vi "findValue.vi"(1 "采集数据":dbl[](array[numeric]), 2 "精度":dbl, 3 "循环点":i32) -> (0 "试验结果":dbl[](array[numeric]))   [LabVIEW 2011]
panel:
  out "内部变量":i32
  out "Numeric":dbl
  out "标志":bool
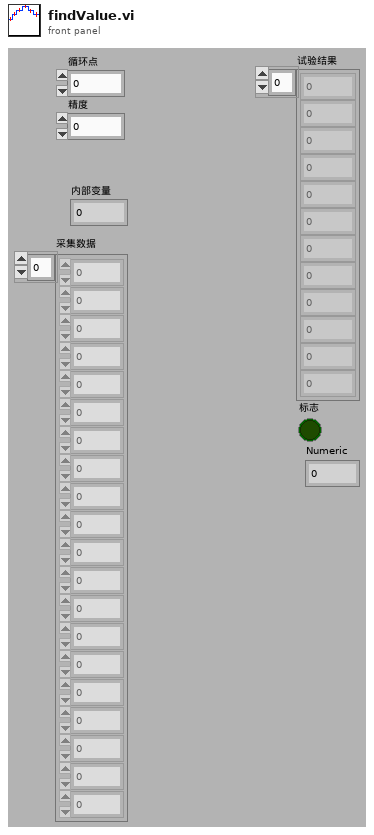
[diagram p1: front panel]
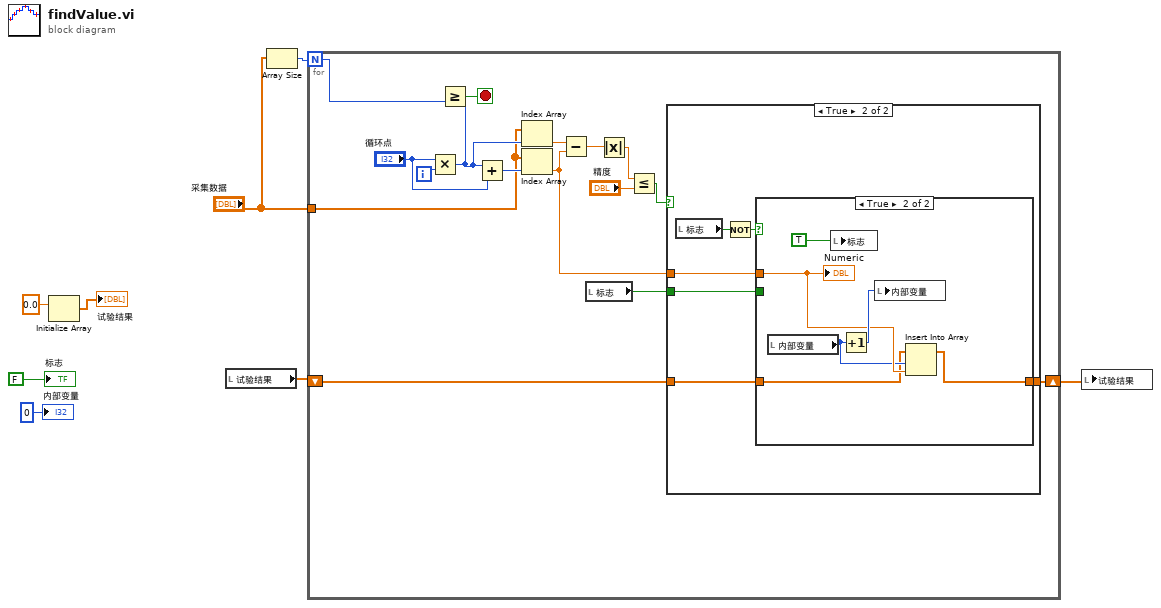
[diagram p0: block diagram]
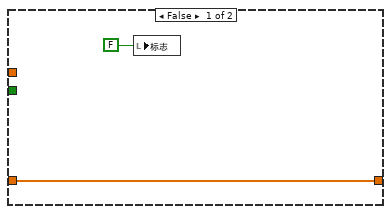
[diagram p2: hidden frame]
diagram:
  n1 = Initialize Array(0.0 ("element")) -> (→"试验结果":dbl[])  [unwired: 1 out]
  n2 = local read "试验结果"() -> (w4:dbl[])
  n3 = Array Size(array="采集数据") -> (size(s)=w7:i32)
  n4 = for {
    N: w7 -> [w23]
    tunnel: "采集数据" -> [w16]
    shift-right: [w9] -> w3
    shift-left: w4 -> [w10]
    i -> [w24]
    stop <- w22 stop-if-true
    n5 = Multiply(x="循环点", y=w24) -> (x*y=w17:i32)
    n6 = Greater Or Equal?(x=w17, y=w23) -> (x >= y?=w22:bool)
    n7 = Add(x=w17, y="循环点") -> (x+y=w18:i32)
    n8 = Index Array(array=w16, index=w17) -> (element=w15:dbl)
    n9 = Index Array(array=w16, index=w18) -> (element=w11:dbl)
    n10 = Subtract(x=w15, y=w11) -> (x-y=w14:dbl)
    n11 = local read "标志"() -> (w12:bool)
    n12 = Absolute Value(x=w14) -> (abs(x)=w13:dbl)
    n13 = Less Or Equal?(x=w13, y="精度") -> (x <= y?=w20:bool)
    n14 = case shown="True" w20 {
      tunnel: w12 -> [_ w30]
      tunnel: w11 -> [_ w29]
      tunnel: w10 -> [w25 w28]
      tunnel: [w25 w27] -> w9
      frame False {
        n15 = local write "标志"(FALSE ("标准")) -> ()
      }
      frame True {
        n16 = local read "标志"() -> (w32:bool)
        n17 = Not(x=w32) -> (.not. x?=w31:bool)
        n18 = case shown="True" w31 {
          tunnel: w30 -> [_ _]
          tunnel: w29 -> [_ w37]
          tunnel: w28 -> [w33 w35]
          tunnel: [w33 w34] -> w27
          frame False {
          }
          frame True {
            n19 = local read "内部变量"() -> (w36:i32)
            n20 = local write "标志"(TRUE ("标准")) -> ()
            n21 = Increment(x=w36) -> (x+1=w38:i32)
            n22 = local write "内部变量"(w38) -> ()
            n23 = Insert Into Array(array=w35, index=w36, new element=w37) -> (w34:dbl[])
            "Numeric" <- w37
          }
        }
      }
    }
  }
  n24 = local write "试验结果"(w3) -> ()
  "标志" <- FALSE ("标准")
  "内部变量" <- 0 ("内部变量")
